vi "Close Shutter.vi"(1 "Channel":i32=1) -> ()   [LabVIEW 2020]
uses:
  Laser Parameters.vi
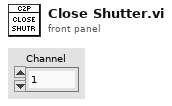
[diagram p1: front panel]
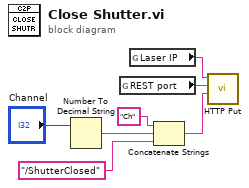
[diagram p0: block diagram]
diagram:
  n1 = Number To Decimal String(number="Channel") -> (decimal integer string=w2:string)  [unwired: 1 in]
  n2 = global read "Laser Parameters.vi" "REST port"() -> (w6:string)
  n3 = global read "Laser Parameters.vi" "Laser IP"() -> (w7:string)
  n4 = Concatenate Strings("Ch" ("Endpoint"), w2, "/ShutterClosed" ("Endpoint")) -> (w4:string)
  n5 = call "HTTP Put.vi"("Endpoint"=w4, "Port"=w6, "IP Address"=w7) -> ()  [unwired: 1 in, 2 out]
